vi "FGV Schedule Daten.vi"(0 "Testreihenfolge:":T1 {"Test 5" items=["---", "Dichtheitstest", "Kalibrieren", "Cal-Gas Test", "T90 Test"]; "Test 4" items=["---", "Dichtheitstest", "Kalibrieren", "Cal-Gas Test", "T90 Test"]; "Test 3" items=["---", "Dichtheitstest", "Kalibrieren", "Cal-Gas Test", "T90 Test"]; "Test 2" items=["---", "Dichtheitstest", "Kalibrieren", "Cal-Gas Test", "T90 Test"]; "Test 1" items=["---", "Dichtheitstest", "Kalibrieren", "Cal-Gas Test", "T90 Test"]}, 1 "Aktive Wochentage":T4, 2 "Zeiten":T5 {"Sonntag" format="%<%H:%M>T"; "Samstag" format="%<%H:%M>T"; "Freitag" format="%<%H:%M>T"; "Donnerstag" format="%<%H:%M>T"; "Mittwoch" format="%<%H:%M>T"; "Dienstag" format="%<%H:%M>T"; "Montag" format="%<%H:%M>T"}, 3 "Planer Status":T3 items=["inaktiv", "aktiv"], 4 "Testreihenfolge AK":T1 {"Test 5" items=["---", "Dichtheitstest", "Kalibrieren", "Cal-Gas Test", "T90 Test"]; "Test 4" items=["---", "Dichtheitstest", "Kalibrieren", "Cal-Gas Test", "T90 Test"]; "Test 3" items=["---", "Dichtheitstest", "Kalibrieren", "Cal-Gas Test", "T90 Test"]; "Test 2" items=["---", "Dichtheitstest", "Kalibrieren", "Cal-Gas Test", "T90 Test"]; "Test 1" items=["---", "Dichtheitstest", "Kalibrieren", "Cal-Gas Test", "T90 Test"]}, 5 "error in (no error)":errorcluster caption="Fehler (Eingang, kein Fehler)", 11 "Aktion":T7) -> (14 "Testreihenfolge:":T1 {"Test 5" items=["---", "Dichtheitstest", "Kalibrieren", "Cal-Gas Test", "T90 Test"]; "Test 4" items=["---", "Dichtheitstest", "Kalibrieren", "Cal-Gas Test", "T90 Test"]; "Test 3" items=["---", "Dichtheitstest", "Kalibrieren", "Cal-Gas Test", "T90 Test"]; "Test 2" items=["---", "Dichtheitstest", "Kalibrieren", "Cal-Gas Test", "T90 Test"]; "Test 1" items=["---", "Dichtheitstest", "Kalibrieren", "Cal-Gas Test", "T90 Test"]}, 15 "Aktive Wochentage":T4, 16 "Zeiten":T5 {"Sonntag" format="%<%H:%M>T"; "Samstag" format="%<%H:%M>T"; "Freitag" format="%<%H:%M>T"; "Donnerstag" format="%<%H:%M>T"; "Mittwoch" format="%<%H:%M>T"; "Dienstag" format="%<%H:%M>T"; "Montag" format="%<%H:%M>T"}, 17 "Planer Status":T3 items=["inaktiv", "aktiv"], 18 "Testreihenfolge AK":T1 {"Test 5" items=["---", "Dichtheitstest", "Kalibrieren", "Cal-Gas Test", "T90 Test"]; "Test 4" items=["---", "Dichtheitstest", "Kalibrieren", "Cal-Gas Test", "T90 Test"]; "Test 3" items=["---", "Dichtheitstest", "Kalibrieren", "Cal-Gas Test", "T90 Test"]; "Test 2" items=["---", "Dichtheitstest", "Kalibrieren", "Cal-Gas Test", "T90 Test"]; "Test 1" items=["---", "Dichtheitstest", "Kalibrieren", "Cal-Gas Test", "T90 Test"]}, 19 "error out":errorcluster caption="Fehler (Ausgang)")   [LabVIEW 2015, in "Schedule Modul.lvlib"]
uses:
  Schedule Modul.lvlib
  Aktion FGV Schedule Daten.ctl
  Testreihenfolge.ctl
  Test-Auswahlfeld.ctl
  Zeitstempel.ctl
  Zeitstempel-Bedienelement.ctl
  Aktive Wochentage.ctl
  Planer Status.ctl
  Allgemein/allgemeine Sub-VIs.lvlib
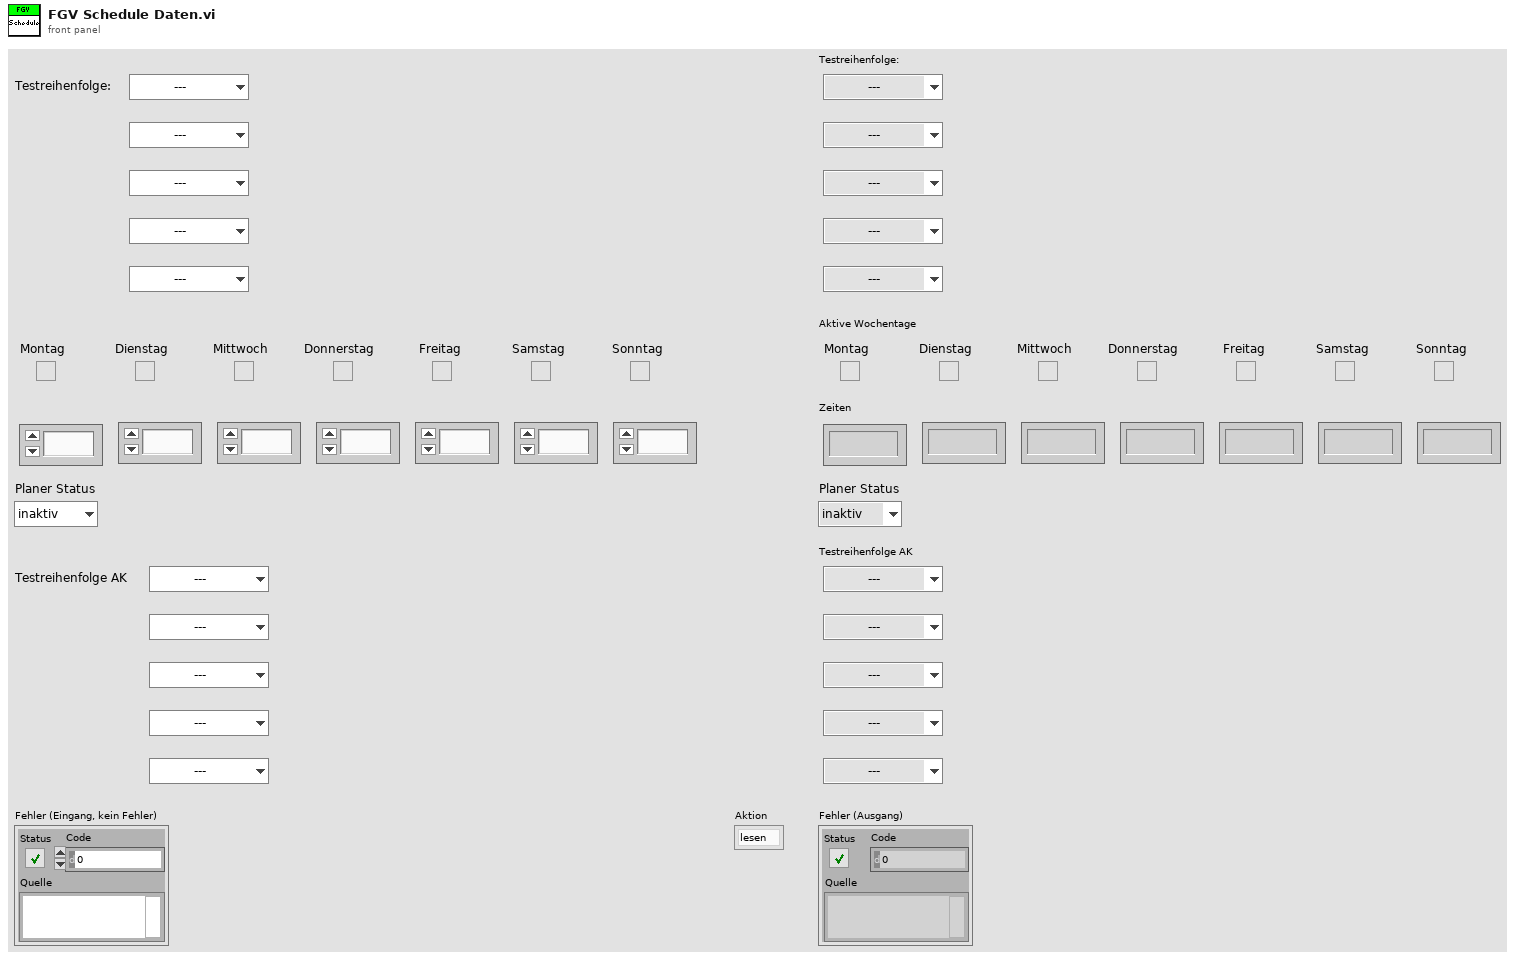
[diagram p1: front panel]
types:
  T1 = typedef "Schedule Modul.lvlib/Testreihenfolge.ctl" = cluster{"Test 1":T2, "Test 2":T2, "Test 3":T2, "Test 4":T2, "Test 5":T2}
  T2 = typedef "Schedule Modul.lvlib/Test-Auswahlfeld.ctl" = u16
  T3 = typedef "Schedule Modul.lvlib/Planer Status.ctl" = u16
  T4 = typedef "Schedule Modul.lvlib/Aktive Wochentage.ctl" = cluster{"Montag":bool, "Dienstag":bool, "Mittwoch":bool, "Donnerstag":bool, "Freitag":bool, "Samstag":bool, "Sonntag":bool}
  T5 = typedef "Schedule Modul.lvlib/Zeitstempel.ctl" = cluster{"Montag":T6, "Dienstag":T6, "Mittwoch":T6, "Donnerstag":T6, "Freitag":T6, "Samstag":T6, "Sonntag":T6}
  T6 = typedef "Schedule Modul.lvlib/Zeitstempel-Bedienelement.ctl" = timestamp
  T7 = typedef "Schedule Modul.lvlib/Aktion FGV Schedule Daten.ctl" = enum16{"lesen", "laden", "speichern", "schreiben"}
  T8 = cluster{"Planer Status":T3, "Zeiten":T5, "Testreihenfolge:":T1, "Aktive Wochentage":T4, "Testreihenfolge AK":T1}
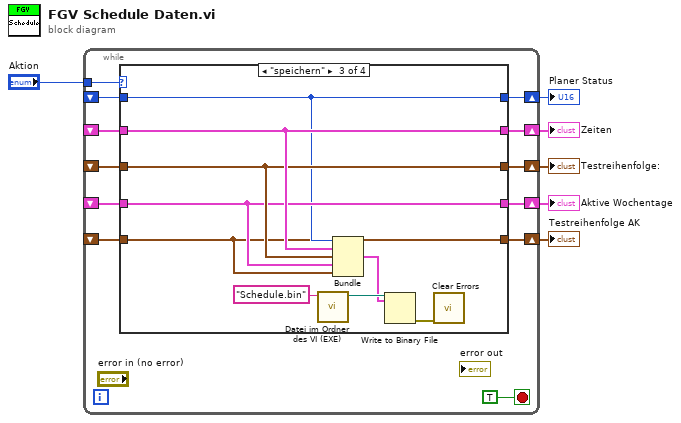
[diagram p0: block diagram]
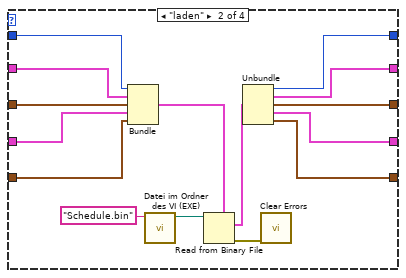
[diagram p3: hidden frame]
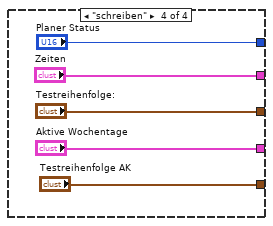
[diagram p4: hidden frame]
diagram:
  n1 = while {
    tunnel: "Aktion" -> [w17]
    shift-right: [w16] -> w5
    shift-left: _ -> [w15]
    shift-right: [w14] -> w4
    shift-left: _ -> [w11]
    shift-right: [w13] -> w3
    shift-left: _ -> [w12]
    shift-right: [w10] -> w2
    shift-left: _ -> [w9]
    shift-right: [w8] -> w1
    shift-left: _ -> [w7]
    stop <- TRUE stop-if-true
    n2 = case shown="\"speichern\"" w17 {
      tunnel: [w23 w27 w47 "Zeiten"] -> w16
      tunnel: w15 -> [w23 w34 w47 _]
      tunnel: [w22 w28 w46 "Testreihenfolge:"] -> w14
      tunnel: w11 -> [w22 w33 w46 _]
      tunnel: [w21 w29 w45 "Aktive Wochentage"] -> w13
      tunnel: w12 -> [w21 w32 w45 _]
      tunnel: [w20 w26 w40 "Planer Status"] -> w10
      tunnel: w9 -> [w20 w30 w40 _]
      tunnel: [w19 w24 w39 "Testreihenfolge AK"] -> w8
      tunnel: w7 -> [w19 w25 w39 _]
      frame "lesen", Default {
      }
      frame "laden" {
        n3 = Bundle("Planer Status"=w30, "Zeiten"=w34, "Testreihenfolge:"=w33, "Aktive Wochentage"=w32, "Testreihenfolge AK"=w25) -> (w31:T8)  [unwired: 1 in]
        n4 = call "Datei im Ordner des VI (EXE).vi"("Dateiname"="Schedule.bin") -> ("Dateipfad im Ordner des Haupt-VIs"=w37:path)  [unwired: 8 in, 2 out]
        n5 = Read from Binary File(5:w31, 11:w37) -> (0:w36:errorcluster, 2:w35:T8)  [unwired: 4 in, 2 out]
        n6 = Unbundle(w35) -> ("Planer Status"=w26:T3, "Zeiten"=w27:T5, "Testreihenfolge:"=w28:T1, "Aktive Wochentage"=w29:T4, "Testreihenfolge AK"=w24:T1)
        n7 = call <vilib>:"Clear Errors.vi"("error in (no error)"=w36) -> ()  [unwired: 5 in, 2 out]
      }
      frame "speichern" {
        n8 = call "Datei im Ordner des VI (EXE).vi"("Dateiname"="Schedule.bin") -> ("Dateipfad im Ordner des Haupt-VIs"=w43:path)  [unwired: 8 in, 2 out]
        n9 = Bundle("Planer Status"=w40, "Zeiten"=w47, "Testreihenfolge:"=w46, "Aktive Wochentage"=w45, "Testreihenfolge AK"=w39) -> (w42:T8)  [unwired: 1 in]
        n10 = Write to Binary File(file (use dialog)=w43, data=w42) -> (error out=w41:errorcluster)  [unwired: 1 in, 5 out]
        n11 = call <vilib>:"Clear Errors.vi"("error in (no error)"=w41) -> ()  [unwired: 5 in, 2 out]
      }
      frame "schreiben" {
      }
    }
  }
  "Zeiten" <- w5
  "Testreihenfolge:" <- w4
  "Aktive Wochentage" <- w3
  "Planer Status" <- w2
  "Testreihenfolge AK" <- w1
